vi "Read Results.vi"(8 "error in (no error)":errorcluster, 11 "Response Synchronizer in":refnum<class "Response Synchronizer.lvclass">) -> (0 "error out":errorcluster, 2 "Results":refnum<class "Acquired Result.lvclass">[](array[class]), 3 "Response Synchronizer out":refnum<class "Response Synchronizer.lvclass">)   [LabVIEW 2021, in "Response Synchronizer.lvclass"]
uses:
  Response Synchronizer.lvclass
  Response Synchronizer.lvclass/Response Synchronizer.ctl
  NHMFL_Core/Libraries/Instruments/Results/Acquired Result/Acquired Result.lvclass
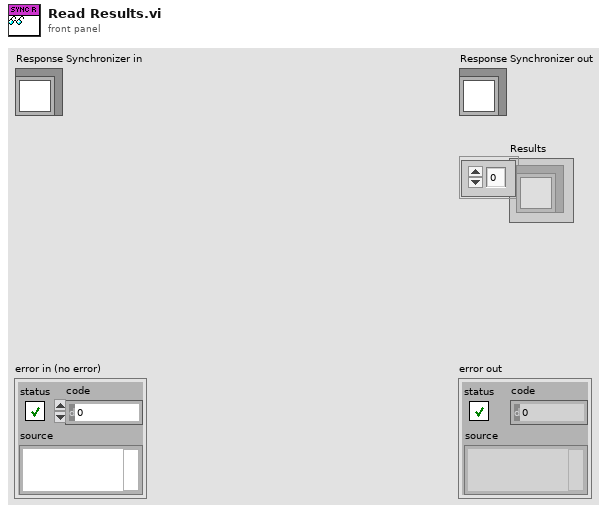
[diagram p1: front panel]
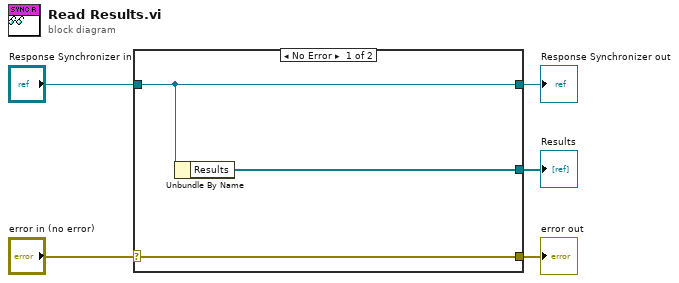
[diagram p0: block diagram]
diagram:
  n1 = case shown="No Error" "error in (no error)" {
    selector: "error in (no error)" -> [w8 w9]
    tunnel: [w8 w9] -> w4
    tunnel: [w7 w10] -> w2
    tunnel: "Response Synchronizer in" -> [w7 w10]
    tunnel: [w6 _] -> w1
    frame No Error {
      n2 = Unbundle By Name(w7) -> ("Results"=w6:refnum<class "Acquired Result.lvclass">[])
    }
    frame Error {
    }
  }
  "error out" <- w4
  "Response Synchronizer out" <- w2
  "Results" <- w1
